vi "High G Graph GUI.vi"(7 "Show last(T)":bool=TRUE, 11 "error in (no error)":errorcluster) -> (15 "error out":errorcluster)   [LabVIEW 2011]
uses:
  Tool/Stroker/High G/high G data GFV Action.ctl
  emi Lib/Basic/0 - General/App/Version/Private/_emi_Version Holder.vi
panel:
  in  "LOAD":bool
  out "Last retrieved High G recording":dbl[][](graph)
  in  "Help":bool
  out "OK":bool
  in  "OK btn":bool
  # "Tab header s can be changed as wanted\n\nCustom can be used for completly ccutom behavior,\nmust then highjack  an other hidden page, for settings"
  # "Add custom behavior taht cvan not be replicated by a simple cluster with valisdity checking"
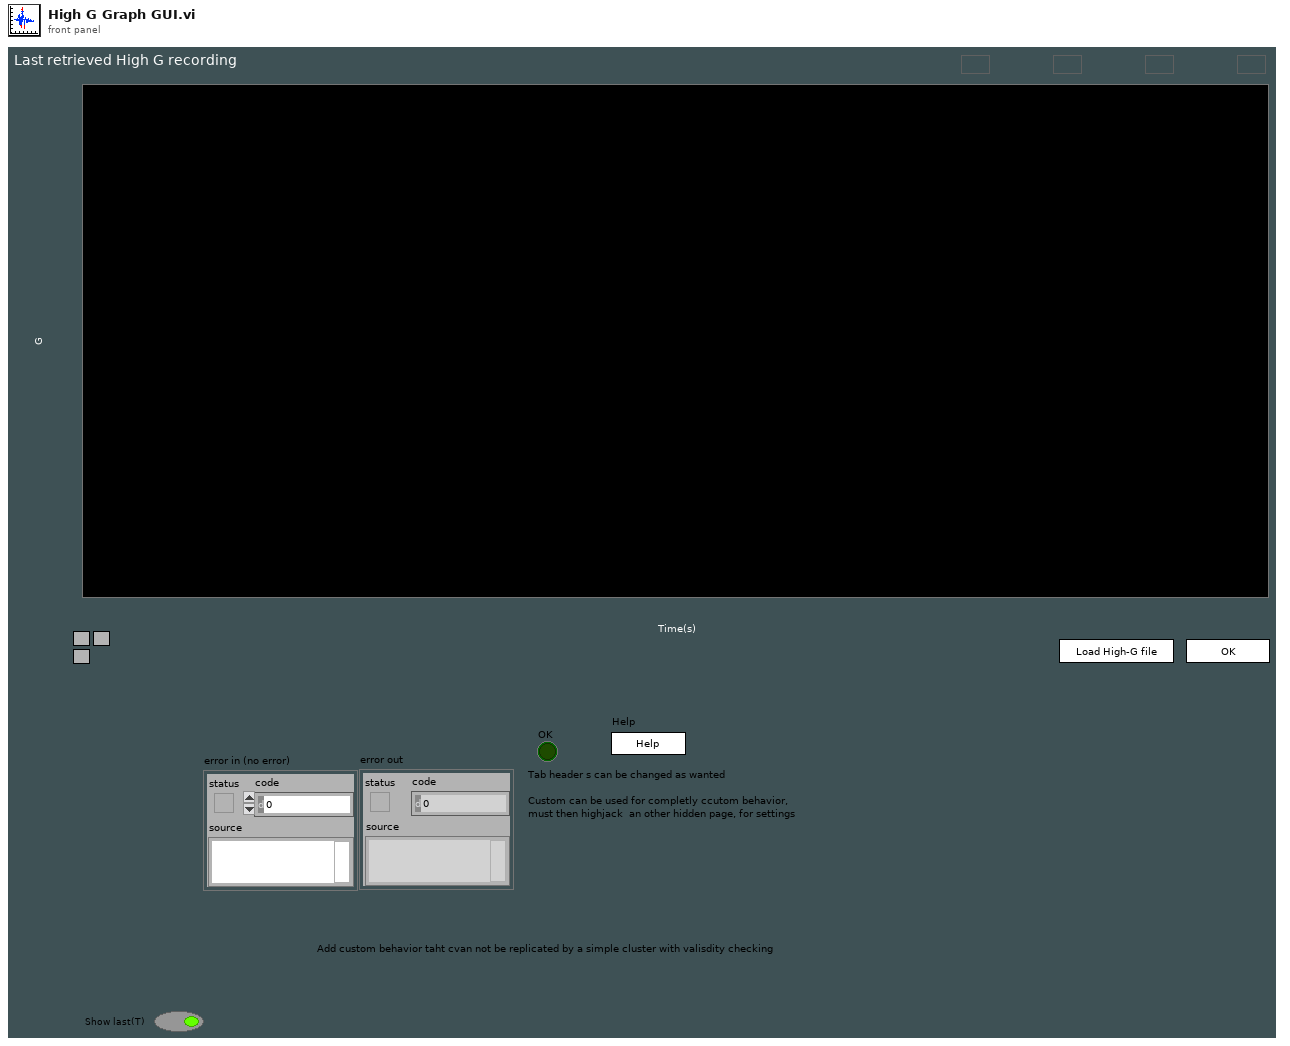
[diagram p1: front panel]
types:
  T1 = typedef "high G data GFV Action.ctl" = enum16{"Init", "Add data", "Get"}
  T2 = typedef "Options  All pages and custom.ctl" = cluster{"P 1 (App)":T3, "P 2":T4, "P 3":T5, "P 4":T8, "P 5":T13, "P 6 (Err)":T14, "P 7 (Expert)":T15, "P 8 (Depth)":T17, "C 1":T18, "C 2":T19}
  T3 = typedef "Options Page 1 (App).ctl" = cluster{"Result files":path, "PCP Interface":string, "Tractor/Stroker Interface":string, "Tractor Interface":string, "Modem Status Interface":string, "Audible Alarm":bool, "Force alarm on Technical":bool, "Force alarm on HH":bool, "Force alarm on LL":bool, "Force alarm on H":bool, "Force alarm on L":bool}
  T4 = typedef "Options Page 2.ctl" = cluster{"Solenoid & Relay latching time":u16, "Tractor relay 1":dbl, "Tractor relay 2":dbl, "Tractor Solenoid limit":dbl}
  T5 = typedef "Options Page 3.ctl" = cluster{"Min resistance":dbl, "Max resistance":dbl, "Head voltage range":T6, "Max voltage jump":dbl, "Maximum resistance change":dbl, "Start Telemetry Voltage":dbl, "Start Telemetry Timeout":dbl, "Start Motor Voltage":dbl, "Stop Motor Voltage":dbl, "Pass Mode Warning Voltage":dbl, "Relay Switch Voltage":dbl, "Relay Status Loss Voltage":dbl, "Samples to average":i32, "PSU type DO NOT USE":T7, "Magna OVP":dbl, "Magna Current Limit":dbl}
  T6 = typedef "PCP type List.ctl" = enum16{"0 - 350V", "0 - 450V", "0 - 600V"}
  T7 = typedef "PSU Type.ctl" = enum16{"Unipower", "Magna 8.3A", "Magna 12A", "None"}
  T8 = typedef "Options Page 4.ctl" = cluster{"Solenoid & Relay latching time":u16, "Stroker relay 1":dbl, "Stroker Relay 2":dbl, "Stroker Solenoid limit":dbl, "Force det.":T9, "Stroke force lim.":dbl, "Anchor Enabled Pressure":dbl, "Tacometer puls":dbl, "Default anchor behavior":T10, "Default stroker behavior":T11, "Default stroker force limit (tonne)":dbl, "Slips Size":T12}
  T9 = typedef "Stroke force selector.ctl" = enum16{"Stroke in = node 1", "Strok out = node 1"}
  T10 = typedef "Default anchor behavior.ctl" = enum16{"Do nothing", "Set Anchor", "Release Anchor"}
  T11 = typedef "Default stroker behavior.ctl" = enum16{"Do nothing", "Stop", "Go Out", "Go In"}
  T12 = typedef "Slips Type Radio.ctl" = enum32{"No Selection", "338 MRS", "3,9 MRS"}
  T13 = typedef "Options Page 5.ctl" = cluster{"Solenoid & Relay latching time":u16, "Driller relay 1":dbl, "Driller Relay 2":dbl, "Driller  Solenoid limit":dbl}
  T14 = typedef "Options Page 6 (Err).ctl" = cluster{"Error and event files":path}
  T15 = typedef "Options Page 7 (Expert).ctl" = cluster{"Show Debug":bool, "Log debug messages":bool, "Additional debug messages":bool, "Start Beagle with Simulator data":bool, "Workshop mode":bool, "Modem baud":u16, "enumCANCOM":bool, "Modem sim":T16, "Telemetry Timeout Disable":i32, "Buffer size":i32, "Upd regular data":bool, "Cable comp":cluster{"VMOD1 Voltage(V)":dbl, "VMOD2 Voltage(V)":dbl}}
  T16 = typedef "Modem simulation setup.ctl" = cluster{"Modem dealay sim":bool, "Sim baud Tx":u16, "Bit Error fraction Tx":dbl, "Sim baud Rx":u16, "Bit Error fraction Rx":dbl}
  T17 = typedef "Options Page 8 (Depth).ctl" = cluster{"Winch Spool Circumference":dbl, "Winch Pulses per Revolution":dbl, "Current Depth":dbl}
  T18 = typedef "Options Custom 1.ctl" = cluster{"Depth Updated":bool, "Depth Offset":dbl}
  T19 = typedef "Options Custom 2.ctl" = cluster{"Placeholder":bool}
  T20 = typedef "emi_Version Info.ctl" = cluster{"Name":string, "Major":i16, "Minor":i16, "Fix":i16, "Build":i32, "Type":enum16{"Alfa", "Beta", "Stable"}, "Dev":bool, "Version Name":string, "Date":timestamp}
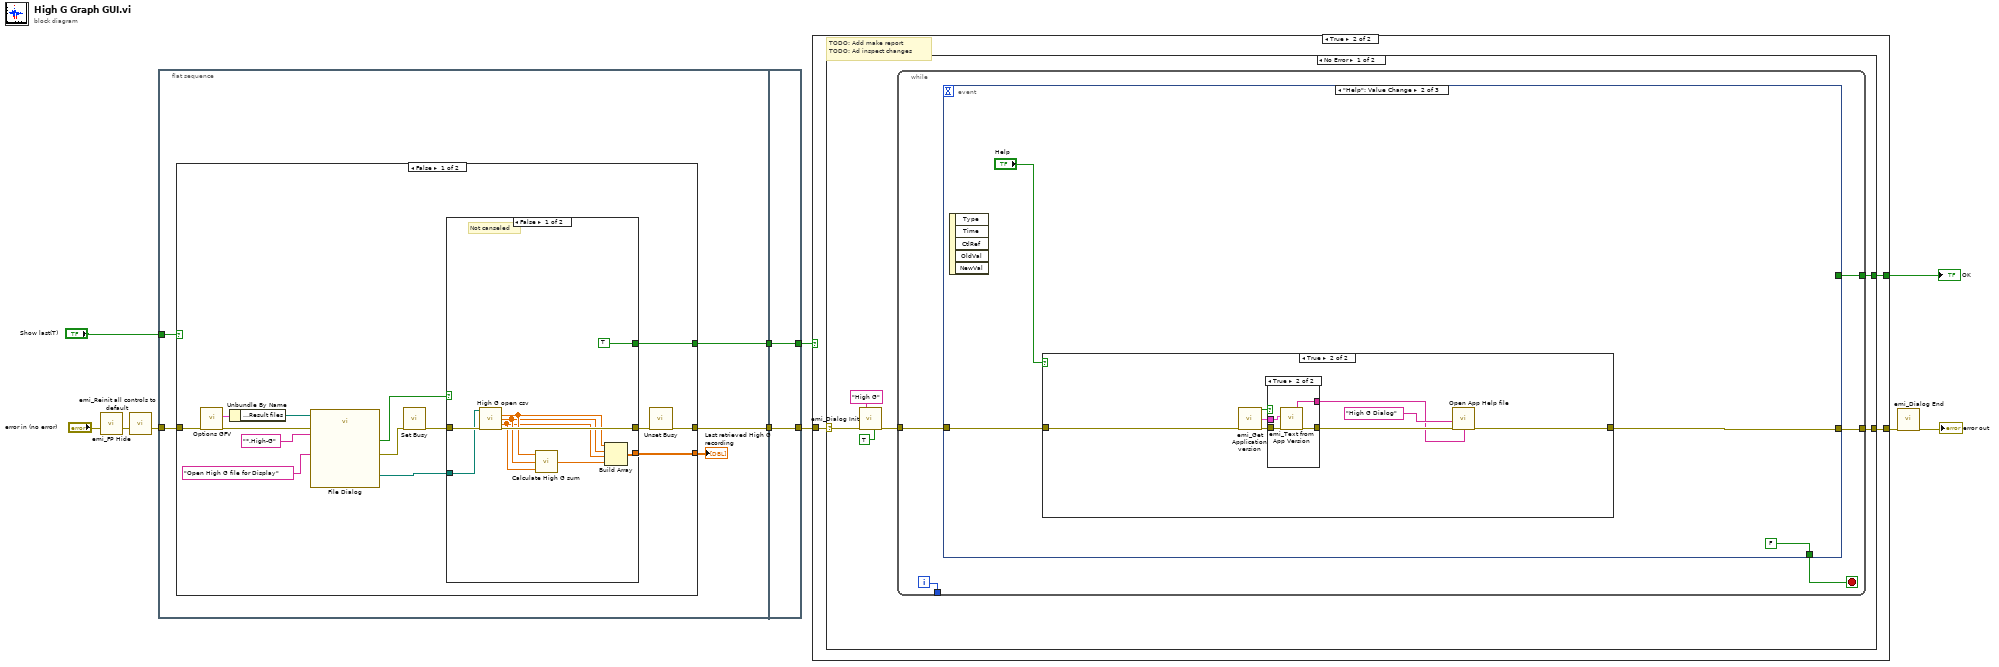
[diagram p0: block diagram]
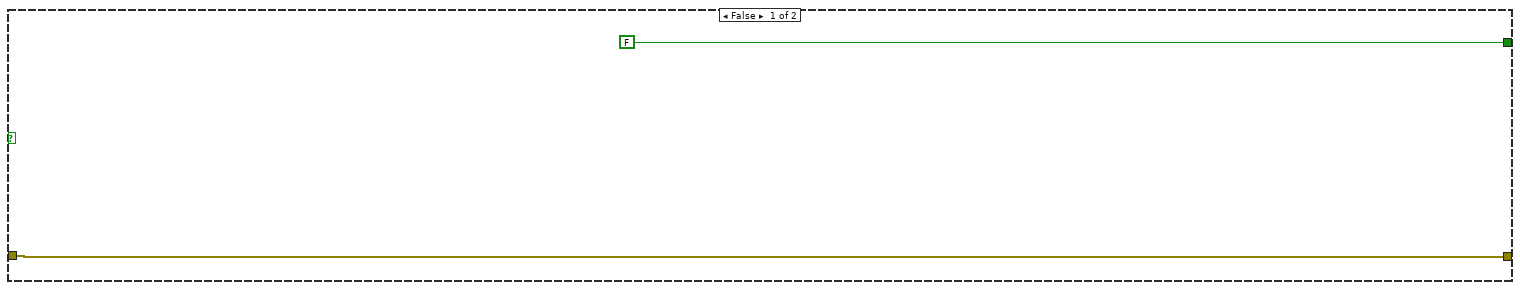
[diagram p2: hidden frame]
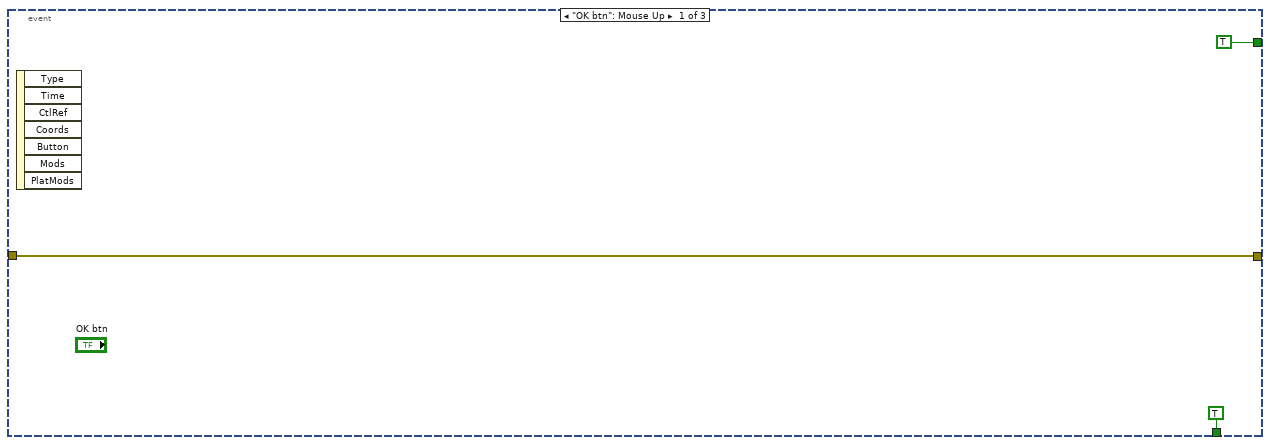
[diagram p3: hidden frame]
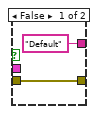
[diagram p5: hidden frame]
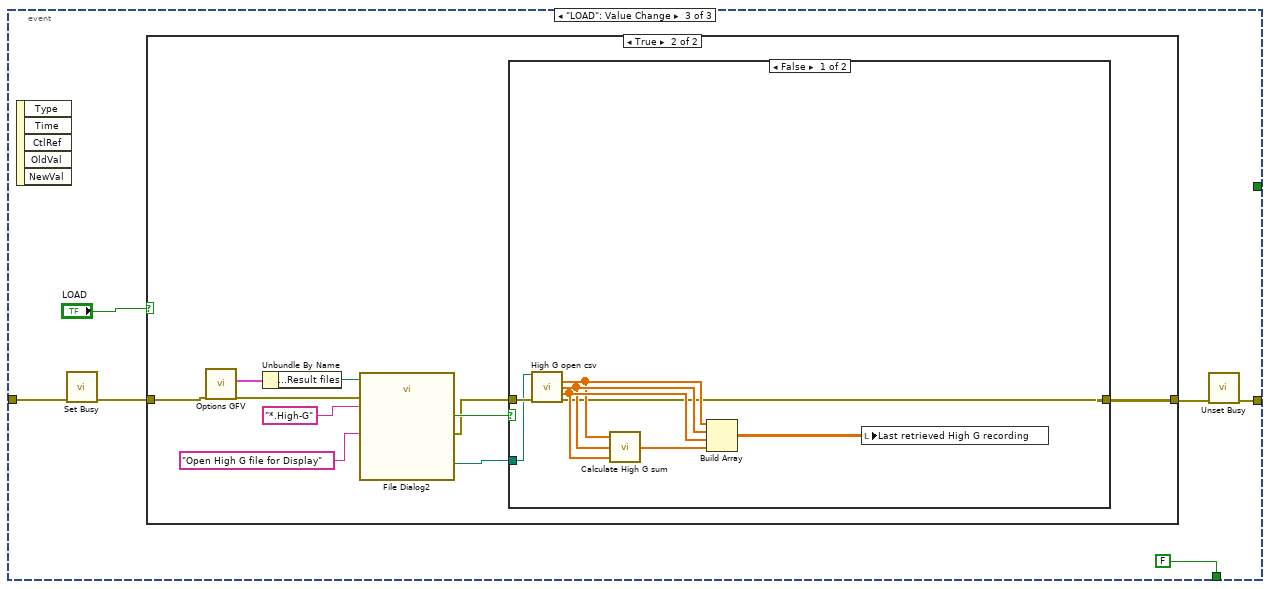
[diagram p6: hidden frame]
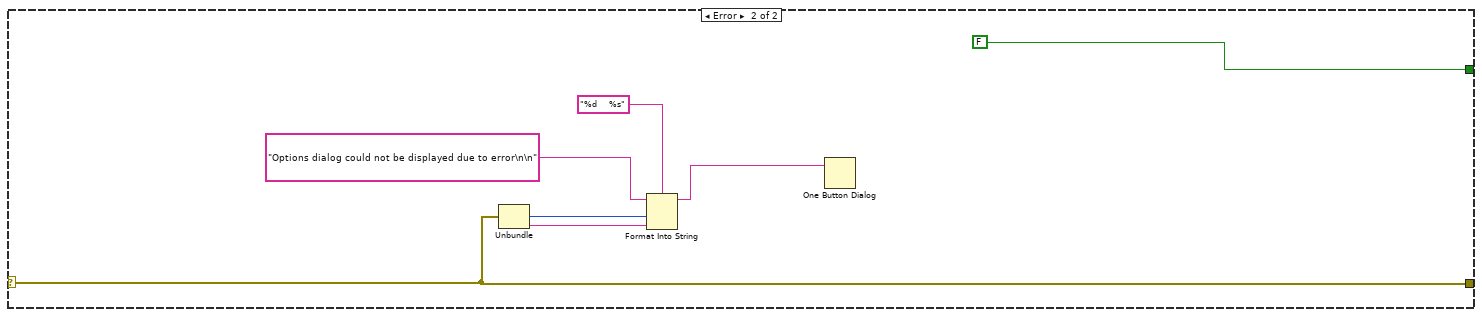
[diagram p9: hidden frame]
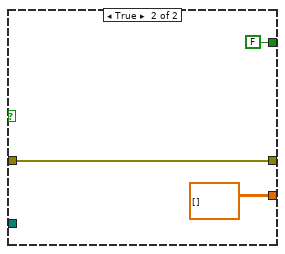
[diagram p10: hidden frame]
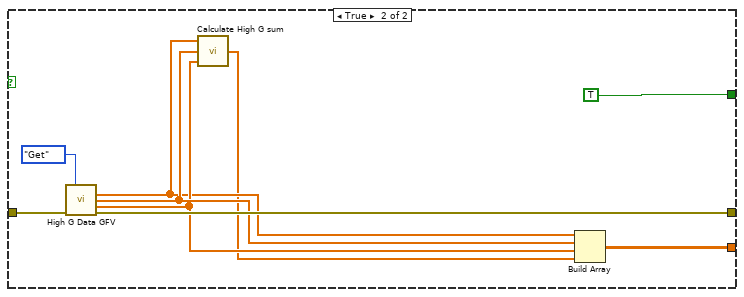
[diagram p11: hidden frame]
diagram:
  n1 = call "emi_FP Hide.vi"("error in (no error)"="error in (no error)") -> ("error out"=w7:errorcluster)  [unwired: 13 in, 1 out]
  n2 = call "emi_Reinit all controls to default.vi"("error in (no error)"=w7) -> ("error out"=w4:errorcluster)  [unwired: 13 in, 1 out]
  n3 = flat-sequence {
    tunnel: w4 -> [w16]
    tunnel: [w15] -> w5
    tunnel: "Show last(T)" -> [w13]
    tunnel: [w12] -> w1
    tunnel: [w53] -> w6
    tunnel: w5 -> [w53]
    tunnel: [w52] -> w2
    tunnel: w1 -> [w52]
    frame #0 {
      n4 = case shown="False" w13 {
        tunnel: w16 -> [w30 w51]
        tunnel: [w17 w49] -> w15
        tunnel: [w20 w44] -> w14
        tunnel: [w21 TRUE] -> w12
        frame False {
          n5 = call "Options GFV.vi"("error in (no error)"=w30) -> ("Options"=w29:T2, "error out"=w27:errorcluster)  [unwired: 16 in, 1 out]
          n6 = Unbundle By Name(w29) -> ("P 1 (App).Result files"=w28:path)
          n7 = call "File Dialog"("start path"=w28, "prompt"="Open High G file for Display", "error in"=w27, "pattern (all files)"="*.High-G") -> ("selected path"=w19:path, "cancelled"=w24:bool, "error out"=w22:errorcluster)  [unwired: 8 in, 1 out]
          n8 = call <vilib>:"Set Busy.vi"("error in (no error)"=w22) -> ("error out"=w18:errorcluster)  [unwired: 9 in, 1 out]
          n9 = case shown="False" w24 {
            tunnel: [w37 w42] -> w23
            tunnel: w18 -> [w39 w42]
            tunnel: [TRUE FALSE] -> w21
            tunnel: [w32 dbl[][] []] -> w20
            tunnel: w19 -> [w38 _]
            frame False {
              # "Not canseled"
              n10 = call "High G open csv.vi"("file path"=w38, "error in (no error)"=w39) -> ("X axis"=w35:dbl[], "Y axis"=w34:dbl[], "Z axis"=w33:dbl[], "error out"=w37:errorcluster)  [unwired: 10 in]
              n11 = call "Calculate High G sum.vi"("Z axis"=w33, "Y axis"=w34, "X axis"=w35) -> ("Sum"=w36:dbl[])
              n12 = Build Array(w35, w34, w33, w36) -> (w32:dbl[][])
            }
            frame True {
            }
          }
          n13 = call <vilib>:"Unset Busy.vi"("error in (no error)"=w23) -> ("error out"=w17:errorcluster)  [unwired: 10 in]
        }
        frame True {
          n14 = call "High G Data GFV.vi"("Action"=high_G_data_GFV_Action."Get", "error in (no error)"=w51) -> ("X axis"=w46:dbl[], "Y axis"=w48:dbl[], "Z axis"=w47:dbl[], "error out"=w49:errorcluster)  [unwired: 9 in, 1 out]
          n15 = call "Calculate High G sum.vi"("Z axis"=w47, "Y axis"=w48, "X axis"=w46) -> ("Sum"=w45:dbl[])
          n16 = Build Array(w46, w48, w47, w45) -> (w44:dbl[][])
        }
      }
      "Last retrieved High G recording" <- w14
    }
    frame #1 {
    }
  }
  n17 = case shown="True" w2 {
    tunnel: [FALSE w58] -> w10
    tunnel: [w54 w57] -> w9
    tunnel: w6 -> [w54 w56]
    frame False {
    }
    frame True {
      # "TODO: Add make report\nTODO: Ad inspect changes"
      n18 = case shown="No Error" w56 {
        selector: w56 -> [w59 w123]
        tunnel: [w64 FALSE] -> w58
        tunnel: [w63 w123] -> w57
        frame No Error {
          n19 = call "emi_Dialog Init.vi"("Header String(\"\")"="High G" ("Header String(\"\")"), "error in"=w59, "Modal(T)"=TRUE) -> ("error out"=w62:errorcluster)  [unwired: 12 in]
          n20 = while {
            tunnel: [w69] -> _
            tunnel: w62 -> [w67]
            tunnel: [w66] -> w63
            tunnel: [w65] -> w64
            i -> [w69]
            stop <- w68 stop-if-true
            n21 = event shown="[1] \"Help\": Value Change" {
              selector: _ -> [_ _ _]
              dyn-events: _ -> [_ _ _]
              timeout: _ -> [_ _ _]
              tunnel: [TRUE FALSE FALSE] -> w68
              tunnel: w67 -> [w70 w74 w95]
              tunnel: [w70 w75 w92] -> w66
              tunnel: [TRUE _ _] -> w65
              event "OK btn": Mouse Up {
                n22 = event-data() -> ()  [unwired: 1 in, 7 out]
              }
              event "Help": Value Change {
                n23 = event-data() -> ()  [unwired: 1 in, 5 out]
                n24 = case shown="True" "Help" {
                  tunnel: [w77 w78] -> w75
                  tunnel: w74 -> [w77 w79]
                  frame False {
                  }
                  frame True {
                    n25 = call "emi_Get Application version.vi"("error in (no error)"=w79) -> ("Version has been set"=w83:bool, "Version Info out"=w82:T20, "error out"=w81:errorcluster)  [unwired: 12 in]
                    n26 = case shown="True" w83 {
                      tunnel: w81 -> [w87 w91]
                      tunnel: w82 -> [_ w90]
                      tunnel: [w87 w89] -> w85
                      tunnel: ["Default" w88] -> w80
                      frame False {
                      }
                      frame True {
                        n27 = call "emi_Text from App Version.vi"("Version Info"=w90, "error in (no error)"=w91) -> ("Name"=w88:string, "error out"=w89:errorcluster)  [unwired: 8 in, 8 out]
                      }
                    }
                    n28 = call "Open App Help file.vi"("Help Tag (\"\")"="High G Dialog" ("Help Tag (\"\")"), "error In"=w85, "file name(\"App\".chm)"=w80) -> ("error out"=w78:errorcluster)  [unwired: 12 in]
                  }
                }
              }
              event "LOAD": Value Change {
                n29 = event-data() -> ()  [unwired: 1 in, 5 out]
                n30 = call <vilib>:"Set Busy.vi"("error in (no error)"=w95) -> ("error out"=w93:errorcluster)  [unwired: 9 in, 1 out]
                n31 = case shown="True" "LOAD" {
                  tunnel: [w98 w100] -> w96
                  tunnel: w93 -> [w98 w103]
                  frame False {
                  }
                  frame True {
                    n32 = call "Options GFV.vi"("error in (no error)"=w103) -> ("Options"=w108:T2, "error out"=w106:errorcluster)  [unwired: 16 in, 1 out]
                    n33 = Unbundle By Name(w108) -> ("P 1 (App).Result files"=w107:path)
                    n34 = call "File Dialog2"("start path"=w107, "prompt"="Open High G file for Display", "error in"=w106, "pattern (all files)"="*.High-G") -> ("selected path"=w99:path, "cancelled"=w102:bool, "error out"=w101:errorcluster)  [unwired: 8 in, 1 out]
                    n35 = case shown="False" w102 {
                      tunnel: w101 -> [w112 w117]
                      tunnel: [w110 w117] -> w100
                      tunnel: w99 -> [w111 _]
                      frame False {
                        n36 = call "High G open csv.vi"("file path"=w111, "error in (no error)"=w112) -> ("X axis"=w114:dbl[], "Y axis"=w115:dbl[], "Z axis"=w116:dbl[], "error out"=w110:errorcluster)  [unwired: 10 in]
                        n37 = call "Calculate High G sum.vi"("Z axis"=w116, "Y axis"=w115, "X axis"=w114) -> ("Sum"=w113:dbl[])
                        n38 = Build Array(w114, w115, w116, w113) -> (w109:dbl[][])
                        n39 = local write "Last retrieved High G recording"(w109) -> ()
                      }
                      frame True {
                        # "Canceled"
                      }
                    }
                  }
                }
                n40 = call <vilib>:"Unset Busy.vi"("error in (no error)"=w96) -> ("error out"=w92:errorcluster)  [unwired: 10 in]
              }
            }
          }
        }
        frame Error {
          n41 = Unbundle(w123) -> ("code"=w120:i32, "source"=w119:string)  [unwired: 1 out]
          n42 = Format Into String(format string="%d    %s", initial string="Options dialog could not be displayed due to error\n\n" ("message"), w120, w119) -> (resulting string=w121:string)  [unwired: 1 in, 1 out]
          n43 = One Button Dialog(message=w121) -> ()  [unwired: 1 in, 1 out]
        }
      }
    }
  }
  "OK" <- w10
  n44 = call "emi_Dialog End.vi"("error in"=w9) -> ("error out"=→"error out":errorcluster)  [unwired: 14 in]
